vi "prepareLogParameters.vi"(8 "error in (no error)":errorcluster, 11 "TestDataLog in":refnum<class "TestDataLog.lvclass">) -> (0 "error out":errorcluster, 2 "LogParameters":string, 3 "TestDataLog out":refnum<class "TestDataLog.lvclass">)   [LabVIEW 2016, in "TestDataLog.lvclass"]
uses:
  TestDataLog.lvclass
  D:/Code/ts_dcabt/Common_Log/Log/Log.lvclass
  Common_Log/Log/Log.lvclass/Log.ctl
  Common_Log/Log/Log.lvclass
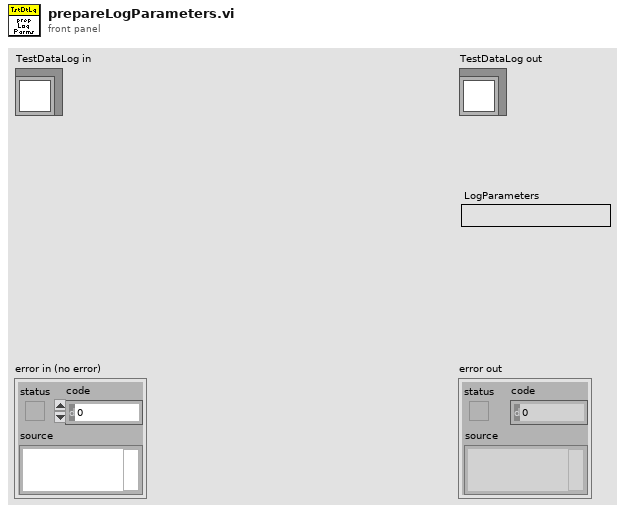
[diagram p1: front panel]
types:
  T1 = typedef "Log.lvlib/Log.ctl" = cluster{"Log Directory":path, "Log Filename Base":string, "Max records per file":u32, "Comment":string}
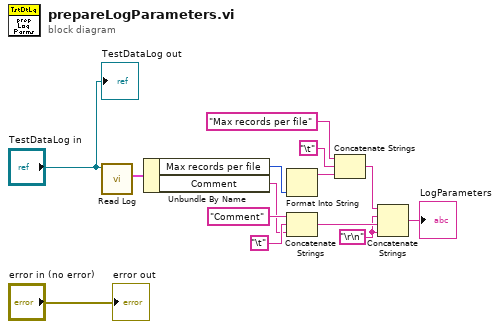
[diagram p0: block diagram]
diagram:
  w3 = "\r\n"
  n1 = call "Read Log.vi"("Log in"="TestDataLog in") -> ("Log"=w13:T1)  [unwired: 9 in, 1 out]
  n2 = Unbundle By Name(w13) -> ("Max records per file"=w12:u32, "Comment"=w6:string)
  n3 = Format Into String(w12) -> (resulting string=w8:string)  [unwired: 3 in, 1 out]
  n4 = Concatenate Strings("Comment" ("element"), "\t", w6) -> (w4:string)
  n5 = Concatenate Strings("Max records per file" ("element"), "\t", w8) -> (w5:string)
  n6 = Concatenate Strings(w5, w3, w4, w3) -> (→"LogParameters":string)
  "error out" <- "error in (no error)"
  "TestDataLog out" <- "TestDataLog in"
